vi "WaitForDigitalIOInputTrigger.vi"(8 "Error In":errorcluster, 9 "Timeout (ms)":u32, 10 "Line (1-14)":u8=1 min=1 max=8 step=1, 11 "Keithley 2602 In":refnum<visa-resource-name>) -> (0 "Error Out":errorcluster, 3 "Keithley 2602 Out":refnum<visa-resource-name>)   [LabVIEW 2012]
uses:
  HardwareAbortGlobalAction.ctl
  driver/Keithley-2602.lvlib
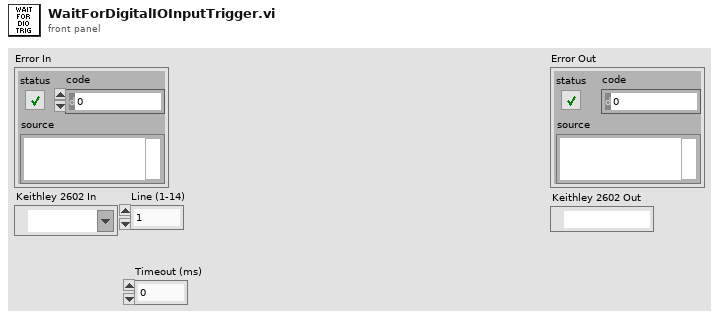
[diagram p1: front panel]
types:
  T1 = typedef "HardwareAbortGlobalAction.ctl" = enum16{"Set", "Get"}
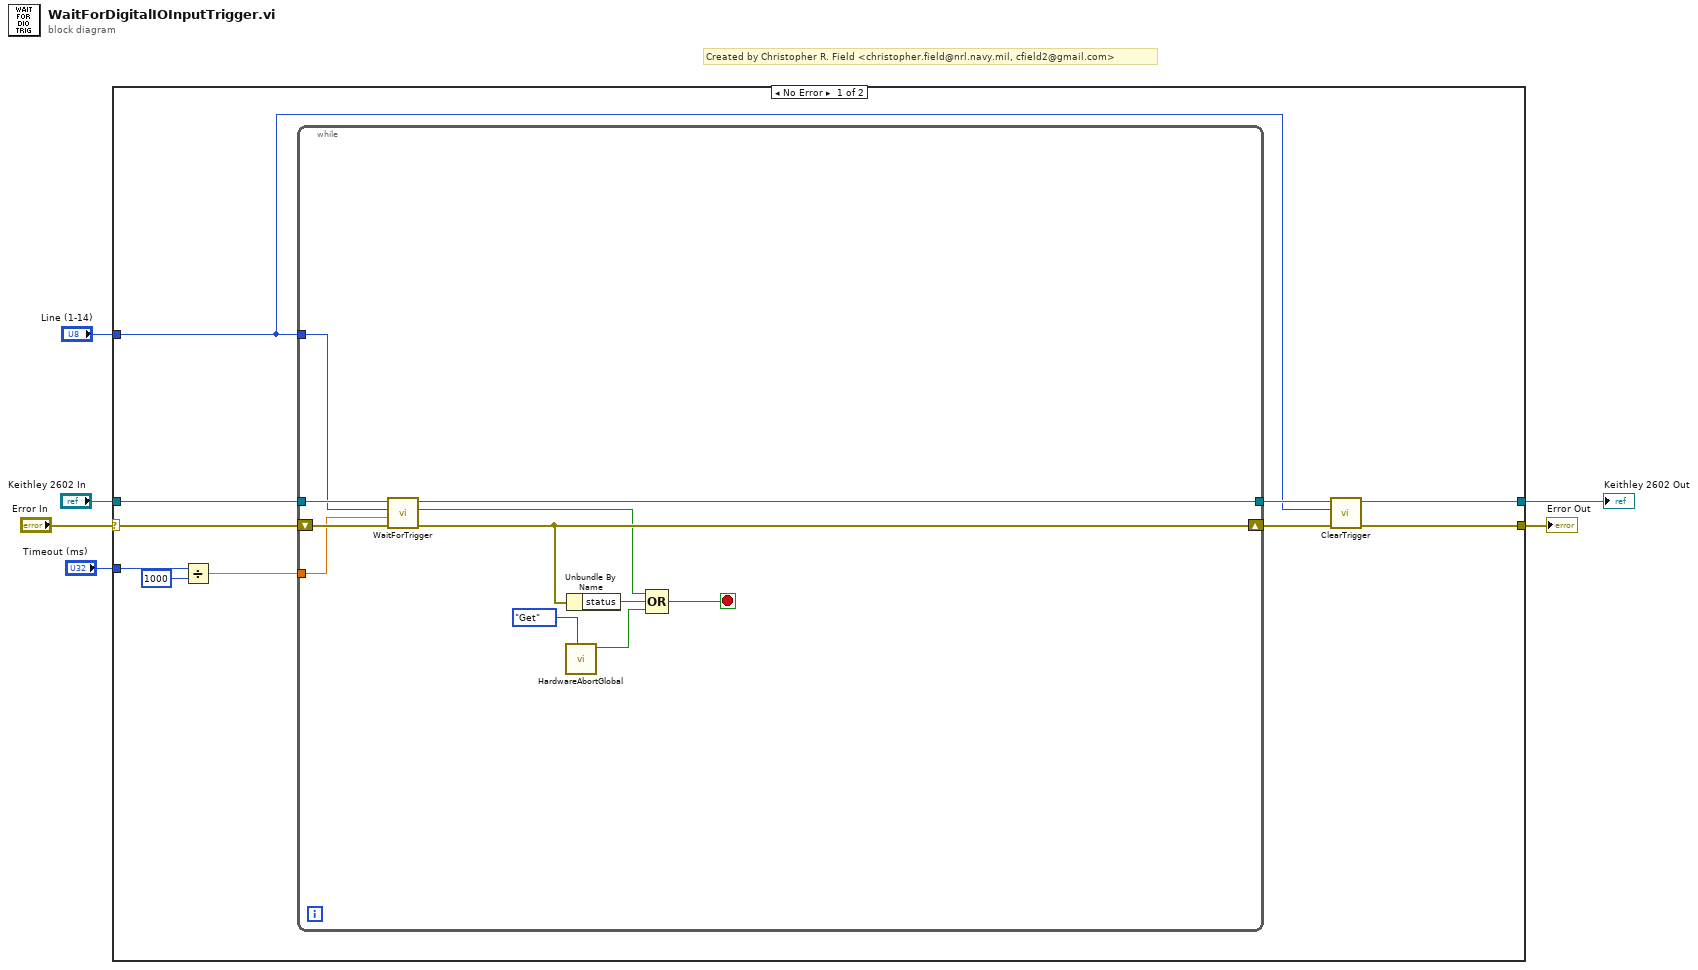
[diagram p0: block diagram]
diagram:
  # "Created by Christopher R. Field <christopher.field@nrl.navy.mil, cfield2@gmail.com>"
  n1 = case shown="No Error" "Error In" {
    selector: "Error In" -> [w16 w28]
    tunnel: [w9 w28] -> w5
    tunnel: "Keithley 2602 In" -> [w15 w29]
    tunnel: [w8 w29] -> w3
    tunnel: "Line (1-14)" -> [w7 _]
    tunnel: "Timeout (ms)" -> [w14 _]
    frame No Error {
      n2 = Divide(x=w14, y=u32 1000) -> (x/y=w12:dbl)
      n3 = while {
        shift-right: [w23] -> w10
        shift-left: w16 -> [w26]
        tunnel: w15 -> [w27]
        tunnel: w7 -> [w25]
        tunnel: [w24] -> w11
        tunnel: w12 -> [w22]
        stop <- w19 stop-if-true
        n4 = call "WaitForTrigger.vi"("Error In"=w26, "Timeout (sec)"=w22, "Line (1-8)"=w25, "Keithley 2602 In"=w27) -> ("Error Out"=w23:errorcluster, "Trigger Detected?"=w21:bool, "Keithley 2602 Out"=w24:refnum<visa-resource-name>)  [unwired: 5 in]
        n5 = call "HardwareAbortGlobal.vi"("Action"=HardwareAbortGlobalAction."Get") -> ("Value Out"=w17:bool)  [unwired: 10 in]
        n6 = Unbundle By Name(w23) -> ("status"=w20:bool)
        n7 = Compound Arithmetic op=OR(w21, w20, w17) -> (w19:bool)
      }
      n8 = call "ClearTrigger.vi"("Error In"=w10, "Line (1-14)"=w7, "Keithley 2602 In"=w11) -> ("Error Out"=w9:errorcluster, "Keithley 2602 Out"=w8:refnum<visa-resource-name>)  [unwired: 7 in]
    }
    frame Error {
    }
  }
  "Error Out" <- w5
  "Keithley 2602 Out" <- w3
